vi "Read PU_CTRL.vi"(8 "error in (no error)":errorcluster, 11 "NAU7802 in":refnum<class "Adafruit NAU7802 24bit Strain Gauge.lvclass">) -> (0 "error out":errorcluster, 2 "Configure NAU7802 CTRL0":T1, 3 "NAU7802 out":refnum<class "Adafruit NAU7802 24bit Strain Gauge.lvclass">)   [LabVIEW 2020, in "CTI-Peripheral.lvlib" / "Adafruit NAU7802 24bit Strain Gauge.lvclass"]
uses:
  Adafruit NAU7802 24bit Strain Gauge.lvclass
  Private/ConfigDataCTRL0.ctl
  Adafruit NAU7802 24bit Strain Gauge.lvclass/Adafruit NAU7802 24bit Strain Gauge.ctl
  CTI/I2C Connection/I2C Connection.lvclass/I2C Connection.ctl
  CTI/Session/I2C Write Data.vi
  CTI/Session/I2C Read Data.vi
  CTI/I2C Connection/I2C Connection.lvclass
panel:
  out "Data":string
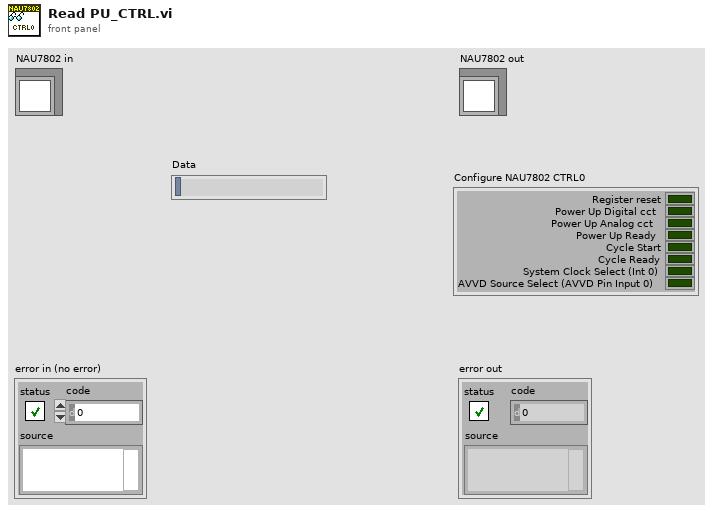
[diagram p1: front panel]
types:
  T1 = typedef "CTI-Peripheral.lvlib/Adafruit NAU7802 24bit Strain Gauge.lvclass/ConfigDataCTRL0.ctl" = cluster{"Register reset":bool, "Power Up Digital cct":bool, "Power Up Analog cct":bool, "Power Up Ready":bool, "Cycle Start":bool, "Cycle Ready":bool, "System Clock Select (Int 0)":bool, "AVVD Source Select (AVVD Pin Input 0)":bool}
  T2 = cluster{"Boolean array[0]":bool, "Boolean array[1]":bool, "Boolean array[2]":bool, "Boolean array[3]":bool, "Boolean array[4]":bool, "Boolean array[5]":bool, "Boolean array[6]":bool, "Boolean array[7]":bool}
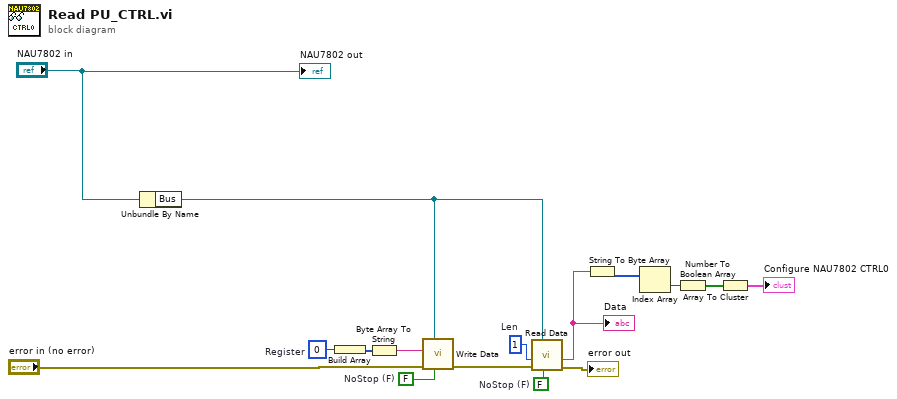
[diagram p0: block diagram]
diagram:
  w7 = u8 0  # Register
  w12 = FALSE  # NoStop (F)
  w13 = u8 1  # Len
  w14 = FALSE  # NoStop (F)
  n1 = Unbundle By Name("NAU7802 in") -> ("Bus"=w11:refnum<class "I2C Connection.lvclass">)
  n2 = Build Array(w7) -> (w8:u8[])
  n3 = Byte Array To String(unsigned byte array=w8) -> (string=w6:string)
  n4 = call "Write Data.vi"("NoStop (F)"=w14, "I2C Connection"=w11, "error in (no error)"="error in (no error)", "Data"=w6) -> ("error out"=w10:errorcluster)  [unwired: 7 in]
  n5 = call "Read Data.vi"("NoStop (F)"=w12, "I2C Connection"=w11, "error in (no error)"=w10, "Len"=w13) -> ("error out"=→"error out":errorcluster, "Data"=w5:string)  [unwired: 6 in]
  "Data" <- w5
  n6 = String To Byte Array(string=w5) -> (unsigned byte array=w4:u8[])
  n7 = Index Array(array=w4) -> (element=w3:u8)  [unwired: 1 in]
  n8 = Number To Boolean Array(number=w3) -> (Boolean array=w2:bool[])
  n9 = Array To Cluster(array=w2) -> (cluster=→"Configure NAU7802 CTRL0":T2)
  "NAU7802 out" <- "NAU7802 in"
